vi "mqttBuildWillinfo.vi"(0 "mqtt in":refnum<class "mqtt.lvclass">, 11 "error in (no error)":errorcluster) -> (4 "mqtt out":refnum<class "mqtt.lvclass">, 8 "willMessage out":u8[](array[numeric]), 15 "error out":errorcluster)   [LabVIEW 2014, in "labview-mqtt.lvlib" / "mqtt.lvclass"]
uses:
  mqtt.lvclass
  mqtt.lvclass/mqtt.ctl
  labview-mqtt.lvlib
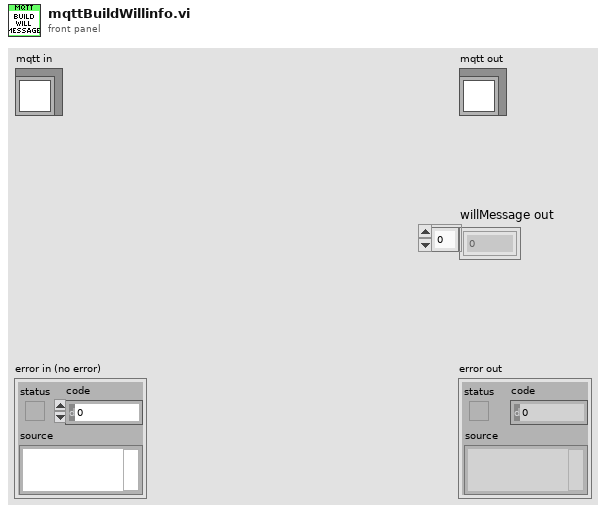
[diagram p1: front panel]
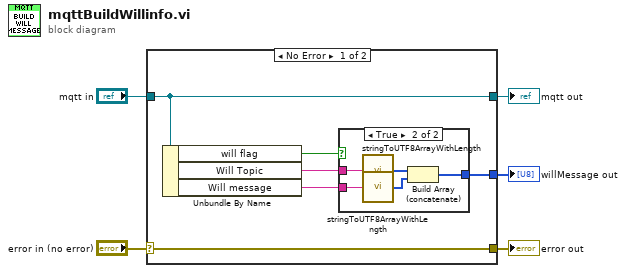
[diagram p0: block diagram]
diagram:
  n1 = case shown="No Error" "error in (no error)" {
    selector: "error in (no error)" -> [w11 w18]
    tunnel: [w11 w18] -> w4
    tunnel: [w10 w17] -> w2
    tunnel: "mqtt in" -> [w10 w17]
    tunnel: [w7 _] -> w1
    frame No Error {
      n2 = Unbundle By Name(w10) -> ("will flag"=w6:bool, "Will Topic"=w8:string, "Will message"=w9:string)
      n3 = case shown="True" w6 {
        tunnel: w9 -> [_ w16]
        tunnel: w8 -> [_ w15]
        tunnel: [_ w12] -> w7
        frame False {
        }
        frame True {
          n4 = call "stringToUTF8ArrayWithLength.vi"("string"=w15) -> ("UTF8[]"=w14:u8[])  [unwired: 14 in]
          n5 = call "stringToUTF8ArrayWithLength.vi"("string"=w16) -> ("UTF8[]"=w13:u8[])  [unwired: 14 in]
          n6 = Build Array (concatenate)(w14, w13) -> (w12:u8[])
        }
      }
    }
    frame Error {
    }
  }
  "error out" <- w4
  "mqtt out" <- w2
  "willMessage out" <- w1
